vi "Load Section - Authentication.vi"(8 "error in (no error)":errorcluster, 11 "JSON string":string) -> (0 "error out":errorcluster, 3 "Class data":refnum<class "Settings Service.lvclass">)   [LabVIEW 2026, in "Settings Service.lvclass"]
uses:
  Settings Service.lvclass
  Settings Service.lvclass/Settings Service.ctl
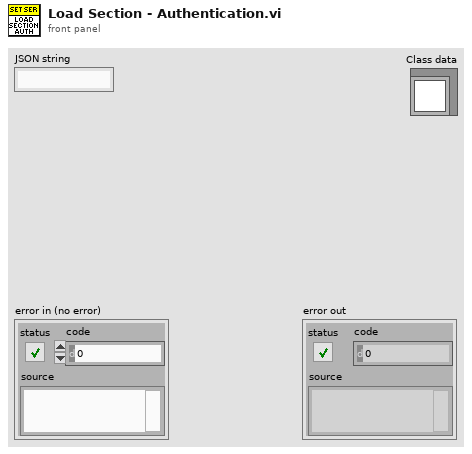
[diagram p1: front panel]
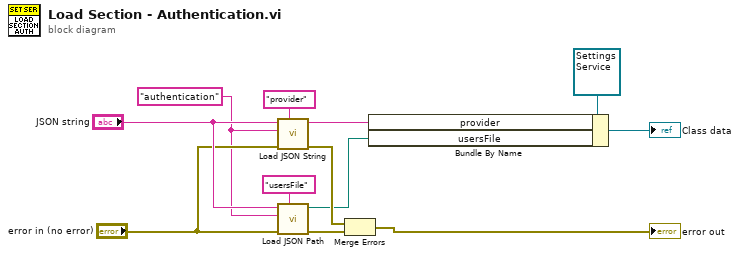
[diagram p0: block diagram]
diagram:
  w9 = "authentication" ("Section")
  n1 = call "Load JSON String.vi"("Element"="provider", "error in (no error)"="error in (no error)", "Section"=w9, "JSON string"="JSON string") -> ("error out"=w7:errorcluster, "value"=w3:string)  [unwired: 6 in]
  n2 = call "Load JSON Path.vi"("Element"="usersFile", "error in (no error)"="error in (no error)", "Section"=w9, "JSON string"="JSON string") -> ("error out"=w6:errorcluster, "value"=w2:path)  [unwired: 6 in]
  n3 = Merge Errors(w7, w6) -> (→"error out":errorcluster)
  n4 = Bundle By Name(cluster=refnum<class "Settings Service.lvclass"> refnum ("Settings Service.lvclass"), "provider"=w3, "usersFile"=w2) -> (→"Class data":refnum<class "Settings Service.lvclass">)
